vi "2Practice.vi"() -> ()   [LabVIEW 2016]
panel:
  in  "file path (use dialog)":path
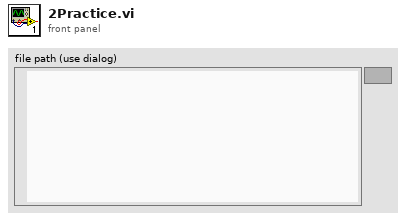
[diagram p1: front panel]
types:
  T1 = enum16{"open", "replace", "create", "open or create", "replace or create", "replace or create with confirmation"}
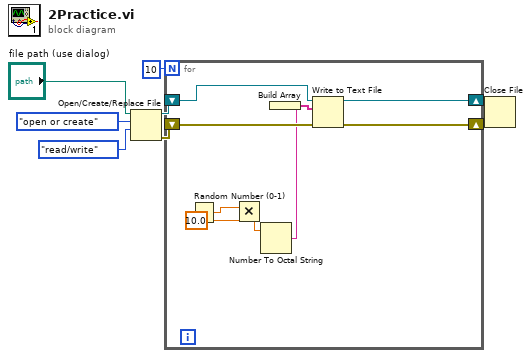
[diagram p0: block diagram]
diagram:
  n1 = Open/Create/Replace File(file path (use dialog)="file path (use dialog)", operation (0:open)=T1."open or create", access (0:read/write)=enum16{"read/write", "read-only", "write-only"}."read/write") -> (refnum out=w3:refnum<file>, error out=w2:errorcluster)  [unwired: 3 in, 1 out]
  n2 = for {
    N: 10 -> [_]
    shift-right: [w17] -> w5
    shift-left: w3 -> [w15]
    shift-right: [w16] -> w4
    shift-left: w2 -> [w14]
    n3 = Random Number (0-1)() -> (number: 0 to 1=w11:dbl)
    n4 = Multiply(x=w11, y=10.0) -> (x*y=w9:dbl)
    n5 = Number To Octal String(2:w9) -> (0:w13:string)  [unwired: 1 in]
    n6 = Build Array(w13) -> (w12:string[])
    n7 = Write to Text File(file (use dialog)=w15, text=w12, error in=w14) -> (refnum out=w17:refnum<file>, error out=w16:errorcluster)  [unwired: 1 in, 1 out]
  }
  n8 = Close File(refnum=w5, error in=w4) -> ()  [unwired: 2 out]
